vi "RTS Standard Test Set Time.vi"(8 "Error In":errorcluster, 11 "Internal Moisture Test (511-B111) - 5 Days":T1={"Chamber 1-3"=[{"End Time"=timestamp(3594046716.8947463 s since 1904-01-01), "Start Time"=timestamp(3593614713.19836 s since 1904-01-01), "Door Opening Schedule:"={"Open Door Timer (s)"=12.0, "Delay Time (s)"=695.0, "Close Door Timer (s)"=12.0}, "Enable Door Ops"=TRUE, "Door Openings"=120, "Temp (°F)"=0.0, "Humidity (%)"=0.0, "Voltage (V)"=0.0, "Door Open Sequence:"=enum."", "Door Delay(sec)"=0.0, "Dehum (°F)"=0.0, "Cool (°F)"=0.0}], "Chamber 1-2"=[{"End Time"=timestamp(3594046708.565822 s since 1904-01-01), "Start Time"=timestamp(3593614700.612354 s since 1904-01-01), "Door Opening Schedule:"={"Open Door Timer (s)"=12.0, "Delay Time (s)"=695.0, "Close Door Timer (s)"=12.0}, "Enable Door Ops"=TRUE, "Door Openings"=0, "Temp (°F)"=0.0, "Humidity (%)"=0.0, "Voltage (V)"=0.0, "Door Open Sequence:"=enum."", "Door Delay(sec)"=0.0, "Dehum (°F)"=0.0, "Cool (°F)"=0.0}], "Chamber 1-1"=[{"End Time"=timestamp(3594046691.867131 s since 1904-01-01), "Start Time"=timestamp(3593614687.850203 s since 1904-01-01), "Door Opening Schedule:"={"Open Door Timer (s)"=12.0, "Delay Time (s)"=2800.0, "Close Door Timer (s)"=12.0}, "Enable Door Ops"=TRUE, "Door Openings"=30, "Temp (°F)"=0.0, "Humidity (%)"=0.0, "Voltage (V)"=0.0, "Door Open Sequence:"=enum."", "Door Delay(sec)"=0.0, "Dehum (°F)"=0.0, "Cool (°F)"=0.0}], "Standard Tests 1-1"=enum."511-B111 Internal Moisture"} {"Chamber 1-1"."Start Time" format="%<%X\n%x>T"; "Chamber 1-1"."End Time" format="%<%X\n%x>T"; "Chamber 1-2"."Start Time" format="%<%X\n%x>T"; "Chamber 1-2"."End Time" format="%<%X\n%x>T"; "Chamber 1-3"."Start Time" format="%<%X\n%x>T"; "Chamber 1-3"."End Time" format="%<%X\n%x>T"}) -> (0 "Error Out":errorcluster, 3 "Output":T1={"Chamber 1-3"=[{"End Time"=timestamp(3594046716.8947463 s since 1904-01-01), "Start Time"=timestamp(3593614713.19836 s since 1904-01-01), "Door Opening Schedule:"={"Open Door Timer (s)"=12.0, "Delay Time (s)"=695.0, "Close Door Timer (s)"=12.0}, "Enable Door Ops"=TRUE, "Door Openings"=120, "Temp (°F)"=0.0, "Humidity (%)"=0.0, "Voltage (V)"=0.0, "Door Open Sequence:"=enum."", "Door Delay(sec)"=0.0, "Dehum (°F)"=0.0, "Cool (°F)"=0.0}], "Chamber 1-2"=[{"End Time"=timestamp(3594046708.565822 s since 1904-01-01), "Start Time"=timestamp(3593614700.612354 s since 1904-01-01), "Door Opening Schedule:"={"Open Door Timer (s)"=12.0, "Delay Time (s)"=695.0, "Close Door Timer (s)"=12.0}, "Enable Door Ops"=TRUE, "Door Openings"=0, "Temp (°F)"=0.0, "Humidity (%)"=0.0, "Voltage (V)"=0.0, "Door Open Sequence:"=enum."", "Door Delay(sec)"=0.0, "Dehum (°F)"=0.0, "Cool (°F)"=0.0}], "Chamber 1-1"=[{"End Time"=timestamp(3594046691.867131 s since 1904-01-01), "Start Time"=timestamp(3593614687.850203 s since 1904-01-01), "Door Opening Schedule:"={"Open Door Timer (s)"=12.0, "Delay Time (s)"=2800.0, "Close Door Timer (s)"=12.0}, "Enable Door Ops"=TRUE, "Door Openings"=30, "Temp (°F)"=0.0, "Humidity (%)"=0.0, "Voltage (V)"=0.0, "Door Open Sequence:"=enum."", "Door Delay(sec)"=0.0, "Dehum (°F)"=0.0, "Cool (°F)"=0.0}], "Standard Tests 1-1"=enum."511-B111 Internal Moisture"} {"Chamber 1-1"."Start Time" format="%<%X\n%x>T"; "Chamber 1-1"."End Time" format="%<%X\n%x>T"; "Chamber 1-2"."Start Time" format="%<%X\n%x>T"; "Chamber 1-2"."End Time" format="%<%X\n%x>T"; "Chamber 1-3"."Start Time" format="%<%X\n%x>T"; "Chamber 1-3"."End Time" format="%<%X\n%x>T"})   [LabVIEW 2016]
uses:
  Type Definitions/RTS Door Op Data.ctl
  Type Definitions/RTS Door Ops Client.ctl
  Type Definitions/RTS Door Opening Schedule.ctl
  Type Definitions/RTS Door Ops Sequence.ctl
  Type Definitions/RTS Standard Door Opening Test.ctl
panel:
  out "Chamber 3 Sec":dbl[](array[numeric])
  out "Chamber 2 Sec":dbl[](array[numeric])
  out "Chamber 1 Sec":dbl[](array[numeric])
  in  "Debug":T1={"Chamber 1-3"=[{"End Time"=timestamp(3594046716.8947463 s since 1904-01-01), "Start Time"=timestamp(3593614713.19836 s since 1904-01-01), "Door Opening Schedule:"={"Open Door Timer (s)"=0.0, "Delay Time (s)"=0.0, "Close Door Timer (s)"=0.0}, "Enable Door Ops"=FALSE, "Door Openings"=120, "Temp (°F)"=78.0, "Humidity (%)"=83.0, "Voltage (V)"=120.0, "Door Open Sequence:"=enum."", "Door Delay(sec)"=0.0, "Dehum (°F)"=70.0, "Cool (°F)"=65.0}, {"End Time"=timestamp(0 s since 1904-01-01), "Start Time"=timestamp(0 s since 1904-01-01), "Door Opening Schedule:"={"Open Door Timer (s)"=6.0, "Delay Time (s)"=705.0, "Close Door Timer (s)"=6.0}, "Enable Door Ops"=TRUE, "Door Openings"=0, "Temp (°F)"=90.0, "Humidity (%)"=65.0, "Voltage (V)"=120.0, "Door Open Sequence:"=enum."", "Door Delay(sec)"=0.0, "Dehum (°F)"=84.0, "Cool (°F)"=85.0}, {"End Time"=timestamp(0 s since 1904-01-01), "Start Time"=timestamp(0 s since 1904-01-01), "Door Opening Schedule:"={"Open Door Timer (s)"=6.0, "Delay Time (s)"=705.0, "Close Door Timer (s)"=6.0}, "Enable Door Ops"=TRUE, "Door Openings"=0, "Temp (°F)"=78.0, "Humidity (%)"=83.0, "Voltage (V)"=120.0, "Door Open Sequence:"=enum."", "Door Delay(sec)"=0.0, "Dehum (°F)"=70.0, "Cool (°F)"=65.0}, {"End Time"=timestamp(0 s since 1904-01-01), "Start Time"=timestamp(0 s since 1904-01-01), "Door Opening Schedule:"={"Open Door Timer (s)"=0.0, "Delay Time (s)"=0.0, "Close Door Timer (s)"=0.0}, "Enable Door Ops"=FALSE, "Door Openings"=0, "Temp (°F)"=78.0, "Humidity (%)"=83.0, "Voltage (V)"=120.0, "Door Open Sequence:"=enum."", "Door Delay(sec)"=0.0, "Dehum (°F)"=70.0, "Cool (°F)"=65.0}], "Chamber 1-2"=[{"End Time"=timestamp(3594046708.565822 s since 1904-01-01), "Start Time"=timestamp(3593614700.612354 s since 1904-01-01), "Door Opening Schedule:"={"Open Door Timer (s)"=0.0, "Delay Time (s)"=0.0, "Close Door Timer (s)"=0.0}, "Enable Door Ops"=FALSE, "Door Openings"=0, "Temp (°F)"=78.0, "Humidity (%)"=83.0, "Voltage (V)"=120.0, "Door Open Sequence:"=enum."", "Door Delay(sec)"=0.0, "Dehum (°F)"=70.0, "Cool (°F)"=65.0}, {"End Time"=timestamp(0 s since 1904-01-01), "Start Time"=timestamp(0 s since 1904-01-01), "Door Opening Schedule:"={"Open Door Timer (s)"=6.0, "Delay Time (s)"=705.0, "Close Door Timer (s)"=6.0}, "Enable Door Ops"=TRUE, "Door Openings"=0, "Temp (°F)"=90.0, "Humidity (%)"=65.0, "Voltage (V)"=120.0, "Door Open Sequence:"=enum."", "Door Delay(sec)"=0.0, "Dehum (°F)"=84.0, "Cool (°F)"=85.0}, {"End Time"=timestamp(0 s since 1904-01-01), "Start Time"=timestamp(0 s since 1904-01-01), "Door Opening Schedule:"={"Open Door Timer (s)"=6.0, "Delay Time (s)"=705.0, "Close Door Timer (s)"=6.0}, "Enable Door Ops"=TRUE, "Door Openings"=0, "Temp (°F)"=78.0, "Humidity (%)"=83.0, "Voltage (V)"=120.0, "Door Open Sequence:"=enum."", "Door Delay(sec)"=0.0, "Dehum (°F)"=70.0, "Cool (°F)"=65.0}, {"End Time"=timestamp(0 s since 1904-01-01), "Start Time"=timestamp(0 s since 1904-01-01), "Door Opening Schedule:"={"Open Door Timer (s)"=0.0, "Delay Time (s)"=0.0, "Close Door Timer (s)"=0.0}, "Enable Door Ops"=FALSE, "Door Openings"=0, "Temp (°F)"=78.0, "Humidity (%)"=83.0, "Voltage (V)"=120.0, "Door Open Sequence:"=enum."", "Door Delay(sec)"=0.0, "Dehum (°F)"=70.0, "Cool (°F)"=65.0}], "Chamber 1-1"=[{"End Time"=timestamp(3594046691.867131 s since 1904-01-01), "Start Time"=timestamp(3593614687.850203 s since 1904-01-01), "Door Opening Schedule:"={"Open Door Timer (s)"=0.0, "Delay Time (s)"=0.0, "Close Door Timer (s)"=0.0}, "Enable Door Ops"=FALSE, "Door Openings"=30, "Temp (°F)"=78.0, "Humidity (%)"=83.0, "Voltage (V)"=120.0, "Door Open Sequence:"=enum."", "Door Delay(sec)"=0.0, "Dehum (°F)"=70.0, "Cool (°F)"=65.0}, {"End Time"=timestamp(0 s since 1904-01-01), "Start Time"=timestamp(0 s since 1904-01-01), "Door Opening Schedule:"={"Open Door Timer (s)"=6.0, "Delay Time (s)"=2800.0, "Close Door Timer (s)"=6.0}, "Enable Door Ops"=TRUE, "Door Openings"=0, "Temp (°F)"=90.0, "Humidity (%)"=65.0, "Voltage (V)"=120.0, "Door Open Sequence:"=enum."", "Door Delay(sec)"=0.0, "Dehum (°F)"=84.0, "Cool (°F)"=85.0}, {"End Time"=timestamp(0 s since 1904-01-01), "Start Time"=timestamp(0 s since 1904-01-01), "Door Opening Schedule:"={"Open Door Timer (s)"=6.0, "Delay Time (s)"=2800.0, "Close Door Timer (s)"=6.0}, "Enable Door Ops"=TRUE, "Door Openings"=0, "Temp (°F)"=78.0, "Humidity (%)"=83.0, "Voltage (V)"=120.0, "Door Open Sequence:"=enum."", "Door Delay(sec)"=0.0, "Dehum (°F)"=70.0, "Cool (°F)"=65.0}, {"End Time"=timestamp(0 s since 1904-01-01), "Start Time"=timestamp(0 s since 1904-01-01), "Door Opening Schedule:"={"Open Door Timer (s)"=0.0, "Delay Time (s)"=0.0, "Close Door Timer (s)"=0.0}, "Enable Door Ops"=FALSE, "Door Openings"=0, "Temp (°F)"=78.0, "Humidity (%)"=83.0, "Voltage (V)"=120.0, "Door Open Sequence:"=enum."", "Door Delay(sec)"=0.0, "Dehum (°F)"=70.0, "Cool (°F)"=65.0}], "Standard Tests 1-1"=enum."511-B110 HUT"} {"Chamber 1-1"."Start Time" format="%<%X\n%x>T"; "Chamber 1-1"."End Time" format="%<%X\n%x>T"; "Chamber 1-2"."Start Time" format="%<%X\n%x>T"; "Chamber 1-2"."End Time" format="%<%X\n%x>T"; "Chamber 1-3"."Start Time" format="%<%X\n%x>T"; "Chamber 1-3"."End Time" format="%<%X\n%x>T"}
  # "Freezer"
  # "Cab"
  # "Slide"
  # "Chamber Conditions:"
  # "Chamber Conditions:"
  # "Chamber Conditions:"
  # "Chamber Conditions:"
  # "Chamber Conditions:"
  # "Chamber Conditions:"
  # "Chamber Conditions:"
  # "Chamber Conditions:"
  # "Chamber Conditions:"
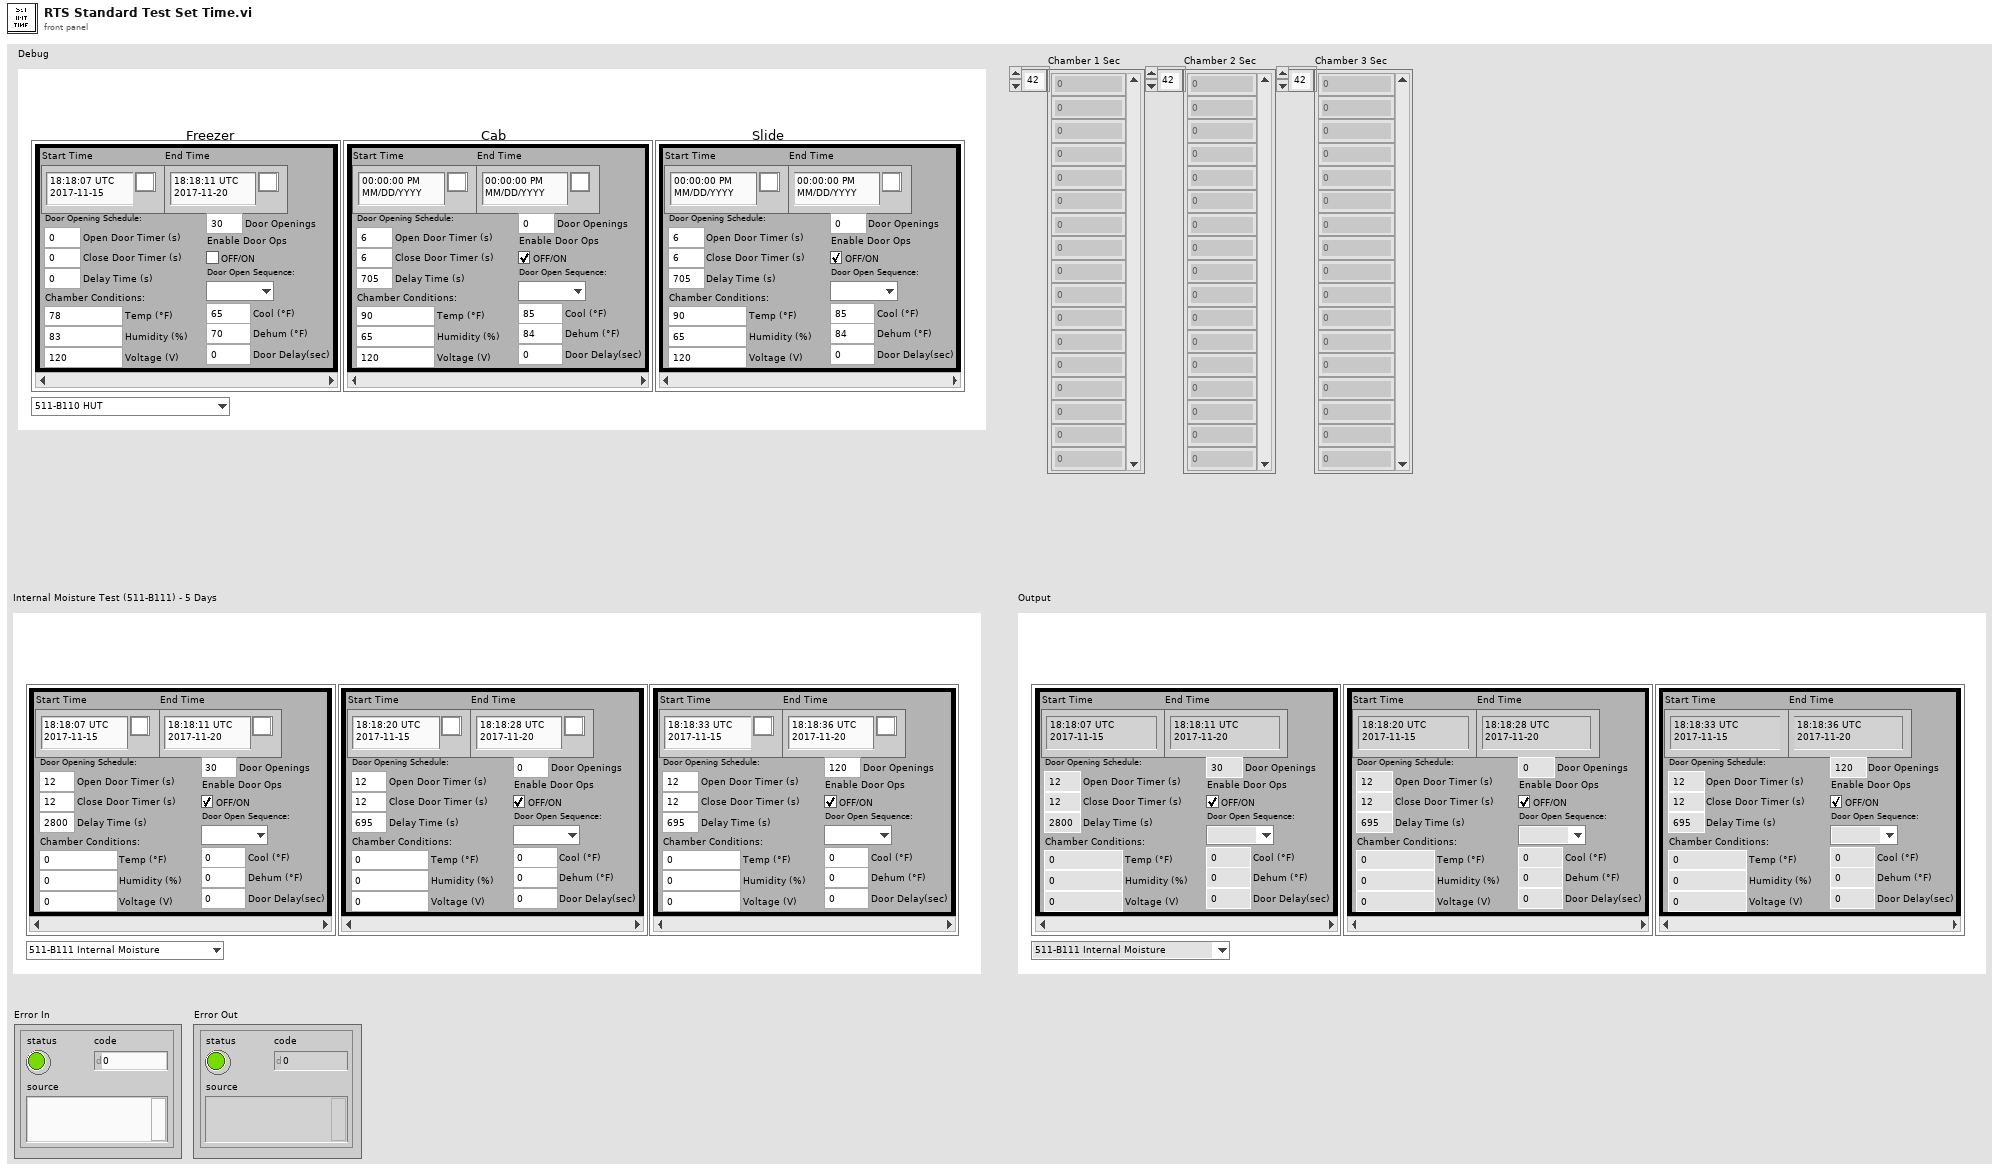
[diagram p1: front panel]
types:
  T1 = typedef "RTS Door Op Data.ctl" = cluster{"Chamber 1-3":T2[], "Chamber 1-2":T2[], "Chamber 1-1":T2[], "Standard Tests 1-1":T5}
  T2 = typedef "RTS Door Ops Client.ctl" = cluster{"End Time":timestamp, "Start Time":timestamp, "Door Opening Schedule:":T3, "Enable Door Ops":bool, "Door Openings":u32, "Temp (°F)":dbl, "Humidity (%)":dbl, "Voltage (V)":dbl, "Door Open Sequence:":T4, "Door Delay(sec)":dbl, "Dehum (°F)":dbl, "Cool (°F)":dbl}
  T3 = typedef "RTS Door Opening Schedule.ctl" = cluster{"Open Door Timer (s)":dbl, "Delay Time (s)":dbl, "Close Door Timer (s)":dbl}
  T4 = typedef "RTS Door Ops Sequence.ctl" = enum16{"", "1st", "2nd", "3rd"}
  T5 = typedef "RTS Standard Door Opening Test.ctl" = enum16{"Standard ETPs", "511-B113 EHUT", "511-B110 HUT", "512-C410 SLAT", "511-B111 Internal Moisture", "511-C401 Moisture Accumulation", "511-B100 No Door Opening (NDO)", "511-B304 ISO Energy Consumption", "Custom Test", "Cancel Test"}
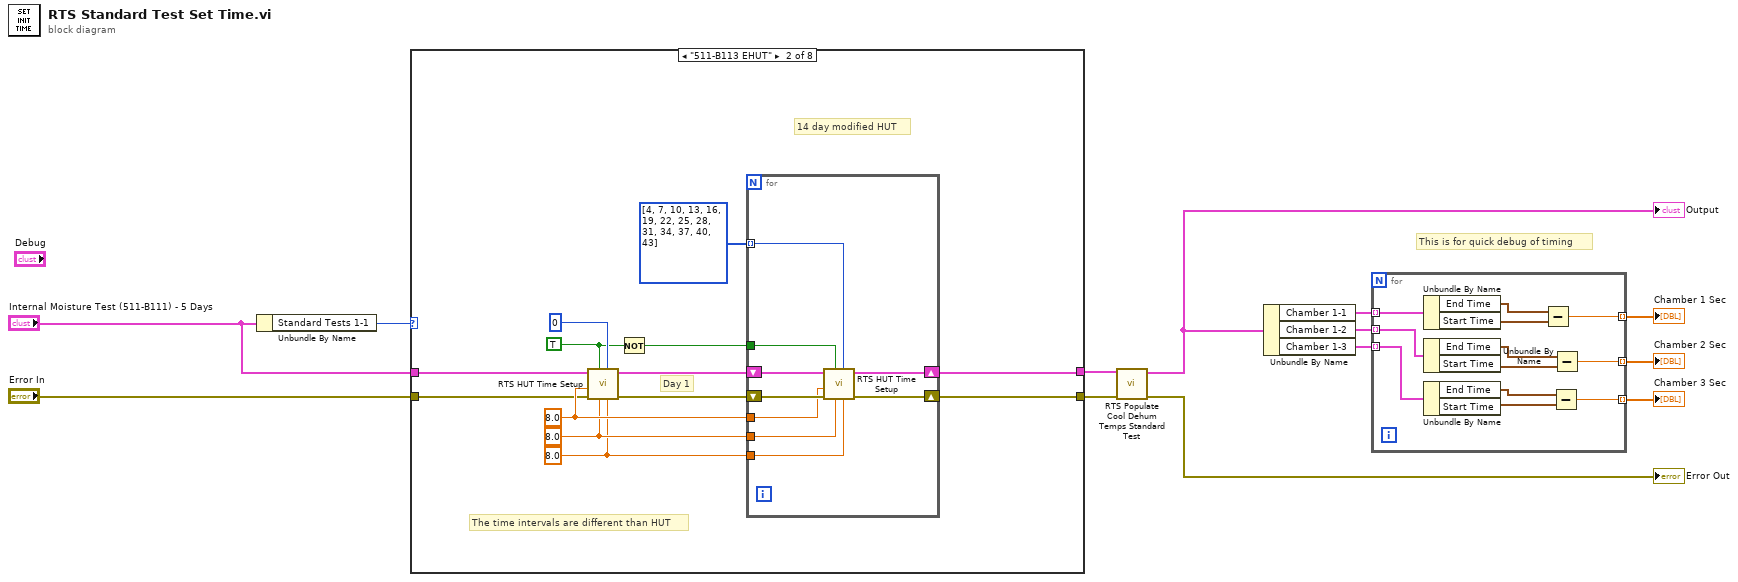
[diagram p0: block diagram]
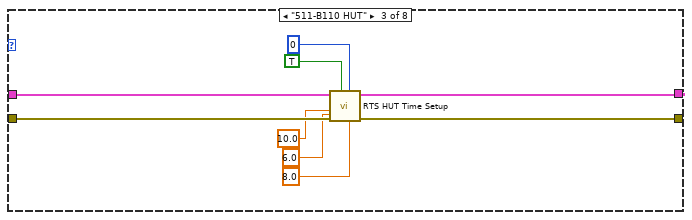
[diagram p3: hidden frame]
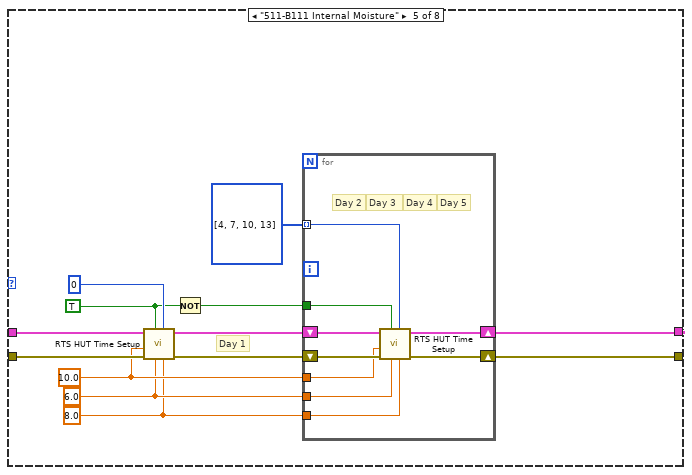
[diagram p5: hidden frame]
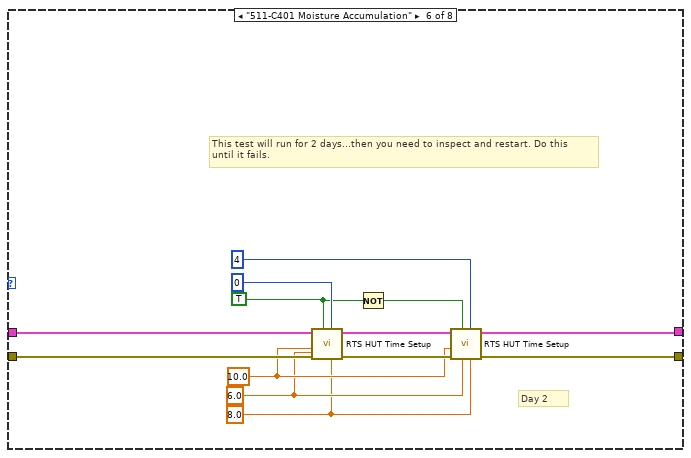
[diagram p6: hidden frame]
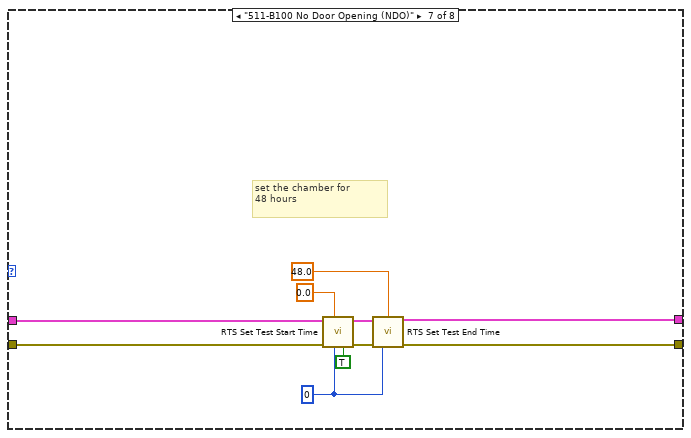
[diagram p7: hidden frame]
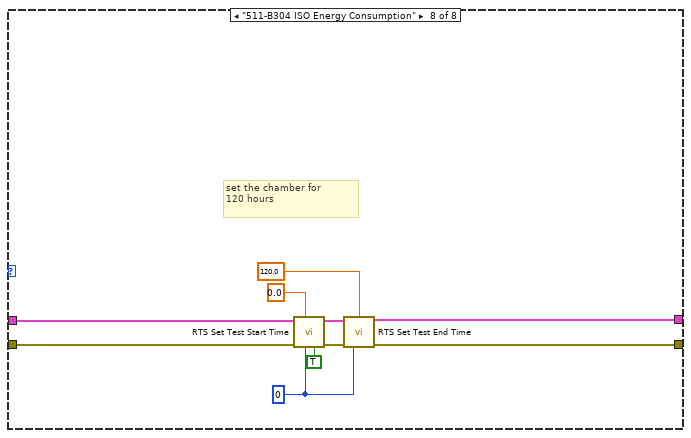
[diagram p8: hidden frame]
diagram:
  # "This is for quick debug of timing"
  n1 = Unbundle By Name("Internal Moisture Test (511-B111) - 5 Days") -> ("Standard Tests 1-1"=w13:T5)
  n2 = case shown="\"511-B113 EHUT\"" w13 {
    tunnel: [w15 w17 w44 w48 w54 w77 w86 w95] -> w4
    tunnel: "Internal Moisture Test (511-B111) - 5 Days" -> [w15 w19 w46 w48 w60 w81 w88 w94]
    tunnel: "Error In" -> [w14 w18 w45 w47 w61 w82 w87 w97]
    tunnel: [w14 w16 w43 w47 w53 w79 w85 w96] -> w3
    frame "Standard ETPs", Default {
    }
    frame "511-B113 EHUT" {
      w20 = 8.0 ("Third Third")
      w21 = 8.0 ("Second Third")
      w22 = 8.0 ("First Third")
      w25 = TRUE ("Pre Condition?")
      # "The time intervals are different than HUT"
      # "14 day modified HUT"
      # "Day 1"
      n3 = call "RTS HUT Time Setup.vi"("Third Third"=w20, "Start Index"=0, "Second Third"=w21, "Pre Condition?"=w25, "error in (no error)"=w18, "First Third"=w22, "Internal Moisture Test (511-B111) - 5 Days"=w19) -> ("error out"=w27:errorcluster, "Current Test Output"=w26:T1)  [unwired: 3 in]
      n4 = Not(x=w25) -> (.not. x?=w24:bool)
      n5 = for {
        tunnel: w24 -> [w35]
        shift-right: [w33] -> w16
        shift-left: w27 -> [w37]
        shift-right: [w34] -> w17
        shift-left: w26 -> [w36]
        tunnel: i32[] [4, 7, 10, 13, 16, 19, 22, 25, 28, 31, 34, 37, 40, 43] -> [w32] mode=indexing
        tunnel: w22 -> [w31]
        tunnel: w21 -> [w30]
        tunnel: w20 -> [w29]
        n6 = call "RTS HUT Time Setup.vi"("Third Third"=w29, "Start Index"=w32, "Second Third"=w30, "Pre Condition?"=w35, "error in (no error)"=w37, "First Third"=w31, "Internal Moisture Test (511-B111) - 5 Days"=w36) -> ("error out"=w33:errorcluster, "Current Test Output"=w34:T1)  [unwired: 3 in]
      }
    }
    frame "511-B110 HUT" {
      n7 = call "RTS HUT Time Setup.vi"("Third Third"=8.0, "Start Index"=0, "Second Third"=6.0, "Pre Condition?"=TRUE, "error in (no error)"=w45, "First Third"=10.0, "Internal Moisture Test (511-B111) - 5 Days"=w46) -> ("error out"=w43:errorcluster, "Current Test Output"=w44:T1)  [unwired: 3 in]
    }
    frame "512-C410 SLAT" {
    }
    frame "511-B111 Internal Moisture" {
      w49 = 8.0 ("Third Third")
      w50 = 6.0 ("Second Third")
      w51 = 10.0 ("First Third")
      w56 = TRUE ("Pre Condition?")
      # "Day 1"
      n8 = call "RTS HUT Time Setup.vi"("Third Third"=w49, "Start Index"=0, "Second Third"=w50, "Pre Condition?"=w56, "error in (no error)"=w61, "First Third"=w51, "Internal Moisture Test (511-B111) - 5 Days"=w60) -> ("error out"=w58:errorcluster, "Current Test Output"=w57:T1)  [unwired: 3 in]
      n9 = Not(x=w56) -> (.not. x?=w55:bool)
      n10 = for {
        tunnel: w55 -> [w68]
        shift-right: [w66] -> w53
        shift-left: w58 -> [w70]
        shift-right: [w67] -> w54
        shift-left: w57 -> [w69]
        tunnel: i32[] [4, 7, 10, 13] -> [w65] mode=indexing
        tunnel: w51 -> [w64]
        tunnel: w50 -> [w63]
        tunnel: w49 -> [w62]
        # "Day 5"
        # "Day 4"
        # "Day 3"
        # "Day 2"
        n11 = call "RTS HUT Time Setup.vi"("Third Third"=w62, "Start Index"=w65, "Second Third"=w63, "Pre Condition?"=w68, "error in (no error)"=w70, "First Third"=w64, "Internal Moisture Test (511-B111) - 5 Days"=w69) -> ("error out"=w66:errorcluster, "Current Test Output"=w67:T1)  [unwired: 3 in]
      }
    }
    frame "511-C401 Moisture Accumulation" {
      w74 = 8.0 ("Third Third")
      w75 = 6.0 ("Second Third")
      w76 = 10.0 ("First Third")
      w73 = TRUE ("Pre Condition?")
      # "This test will run for 2 days...then you need to inspect and restart. Do this \nuntil it fails."
      # "Day 2"
      n12 = call "RTS HUT Time Setup.vi"("Third Third"=w74, "Start Index"=0, "Second Third"=w75, "Pre Condition?"=w73, "error in (no error)"=w82, "First Third"=w76, "Internal Moisture Test (511-B111) - 5 Days"=w81) -> ("error out"=w80:errorcluster, "Current Test Output"=w78:T1)  [unwired: 3 in]
      n13 = Not(x=w73) -> (.not. x?=w72:bool)
      n14 = call "RTS HUT Time Setup.vi"("Third Third"=w74, "Start Index"=4, "Second Third"=w75, "Pre Condition?"=w72, "error in (no error)"=w80, "First Third"=w76, "Internal Moisture Test (511-B111) - 5 Days"=w78) -> ("error out"=w79:errorcluster, "Current Test Output"=w77:T1)  [unwired: 3 in]
    }
    frame "511-B100 No Door Opening (NDO)" {
      w84 = 0 ("index")
      # "set the chamber for\n48 hours"
      n15 = call "RTS Set Test Start Time.vi"("Use Current Time As Start?"=TRUE, "index"=w84, "Start Time Offset"=0.0, "Error In"=w87, "Current Test"=w88) -> ("Error Out"=w92:errorcluster, "Current Test Output"=w93:T1)  [unwired: 5 in]
      n16 = call "RTS Set Test End Time.vi"("Current Test"=w93, "Operation Duration (hrs)"=48.0 ("Operation Duration"), "Error In"=w92, "index"=w84) -> ("Current Test Output"=w86:T1, "Error Out"=w85:errorcluster)  [unwired: 10 in]
    }
    frame "511-B304 ISO Energy Consumption" {
      w98 = 0 ("index")
      # "set the chamber for\n120 hours"
      n17 = call "RTS Set Test Start Time.vi"("Use Current Time As Start?"=TRUE, "index"=w98, "Start Time Offset"=0.0, "Error In"=w97, "Current Test"=w94) -> ("Error Out"=w102:errorcluster, "Current Test Output"=w103:T1)  [unwired: 5 in]
      n18 = call "RTS Set Test End Time.vi"("Current Test"=w103, "Operation Duration (hrs)"=120.0 ("Operation Duration"), "Error In"=w102, "index"=w98) -> ("Current Test Output"=w95:T1, "Error Out"=w96:errorcluster)  [unwired: 10 in]
    }
  }
  n19 = call "RTS Populate Cool Dehum Temps Standard Test.vi"("Error In"=w3, "Current Test Input"=w4) -> ("Error Out"=→"Error Out":errorcluster, "Current Test Output"=w1:T1)  [unwired: 8 in]
  "Output" <- w1
  n20 = Unbundle By Name(w1) -> ("Chamber 1-1"=w10:T2[], "Chamber 1-2"=w9:T2[], "Chamber 1-3"=w8:T2[])
  n21 = for {
    tunnel: w10 -> [w115] mode=indexing
    tunnel: w9 -> [w114] mode=indexing
    tunnel: w8 -> [w113] mode=indexing
    tunnel: [w110] -> w7 mode=indexing
    tunnel: [w107] -> w6 mode=indexing
    tunnel: [w104] -> w5 mode=indexing
    n22 = Unbundle By Name(w115) -> ("End Time"=w112:timestamp, "Start Time"=w111:timestamp)
    n23 = Unbundle By Name(w114) -> ("End Time"=w109:timestamp, "Start Time"=w108:timestamp)
    n24 = Unbundle By Name(w113) -> ("End Time"=w106:timestamp, "Start Time"=w105:timestamp)
    n25 = Subtract(x=w112, y=w111) -> (x-y=w110:dbl)
    n26 = Subtract(x=w106, y=w105) -> (x-y=w104:dbl)
    n27 = Subtract(x=w109, y=w108) -> (x-y=w107:dbl)
  }
  "Chamber 1 Sec" <- w7
  "Chamber 2 Sec" <- w6
  "Chamber 3 Sec" <- w5
